vi "Write Flow Rate.vi"(8 "error in":errorcluster, 10 "Flow Rate":T1, 11 "CPC in":refnum<class "CPC.lvclass">) -> (0 "error out":errorcluster, 3 "CPC out":refnum<class "CPC.lvclass">)   [LabVIEW 2014, in "CPC.lvclass"]
doc: "Set the flow rate on the CPC to either low or high."
uses:
  CPC.lvclass
  Controls/3022A/Enum Cmd.ctl
  3022A/3022A.lvclass
  Controls/CmdStruct.ctl
  Controls/3022A/Flow.ctl
panel:
  out "read buffer":string
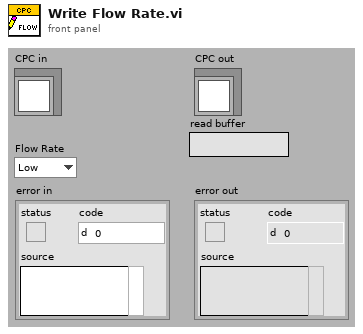
[diagram p1: front panel]
types:
  T1 = typedef "CPC.lvclass/Flow.ctl" = enum16{"Low", "High"}
  T2 = typedef "CmdStruct.ctl" = cluster{"Cmd":u8, "x":i64, "y":i64, "Display":string}
  T3 = typedef "3022A.lvclass/Enum Cmd.ctl" = enum8{"CALIBRATE", "GET CAL DATA", "DUMP", "ESCAPE", "ID CAL LABEL", "INPUT CAL LABEL", "LIQUID LEVEL", "CONDENSER T", "SATURATOR T", "OPTICS T", "GET FLOW RATE", "READ ENV", "READ REF DETECTOR", "READ DETECTOR V", "READ 200 s BUFFER", "READ 20 s BUFFER", "READ 2 s BUFFER", "READ 1 s BUFFER", "READ PHOTOMETRIC CONC", "READ FP CONC", "READ MICROPROCESSOR PUMP CTL", "SENSOR", "SET VOLTAGE", "WRITE DISP MSG", "LASER OFF", "LASER ON", "PUMP OFF", "PUMP ON", "DRAIN", "FILL", "RESET CONC BUFFERS", "LOW FLOW MODE", "HIGH FLOW MODE"}
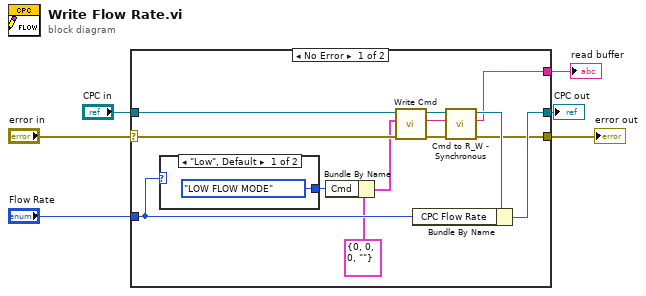
[diagram p0: block diagram]
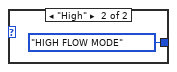
[diagram p2: hidden frame]
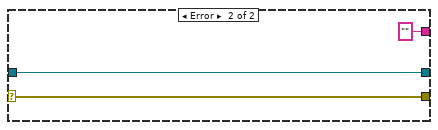
[diagram p3: hidden frame]
diagram:
  n1 = case shown="No Error" "error in" {
    selector: "error in" -> [w16 w23]
    tunnel: [w11 w23] -> w5
    tunnel: [w19 w24] -> w3
    tunnel: "CPC in" -> [w18 w24]
    tunnel: "Flow Rate" -> [w17 _]
    tunnel: [w7 "" ("read buffer")] -> w1
    frame No Error {
      n2 = case shown="\"Low\", Default" w17 {
        tunnel: [Enum_Cmd."LOW FLOW MODE" ("Cmd") Enum_Cmd."HIGH FLOW MODE" ("Cmd")] -> w9
        frame "Low", Default {
        }
        frame "High" {
        }
      }
      n3 = Bundle By Name(cluster=T2 {"Cmd"=0, "x"=0, "y"=0, "Display"=""} ("CmdStruct"), "Cmd"=w9) -> (w8:T2)
      n4 = call-dynamic "Write Cmd.vi"("error in"=w16, "CmdStruct"=w8, "CPC in"=w18) -> ("error out"=w13:errorcluster, "Buffer"=w14:string, "CPC out"=w15:refnum<class "CPC.lvclass">)  [unwired: 6 in]
      n5 = call-dynamic "Cmd to R_W - Synchronous.vi"("error in"=w13, "write buffer"=w14, "Serial IO in"=w15) -> ("error out"=w11:errorcluster, "read buffer"=w7:string, "Serial IO out"=w12:refnum<class "CPC.lvclass">)  [unwired: 6 in]
      n6 = Bundle By Name(cluster=w12, "CPC Flow Rate"=w17) -> (w19:refnum<class "CPC.lvclass">)
    }
    frame Error {
    }
  }
  "error out" <- w5
  "CPC out" <- w3
  "read buffer" <- w1
